vi "Equals.vi"(8 "error in (no error)":errorcluster caption="错误输入（无错误）", 10 "Point 输入":refnum<class "Point.lvclass"> caption="DNL_LabVIEW Object in", 11 "Point 输入":refnum<class "Point.lvclass"> caption="DNL_LabVIEW Object in") -> (0 "error out":errorcluster caption="错误输出", 2 "Equals":bool, 3 "Point 输出":refnum<class "Point.lvclass"> caption="DNL_LabVIEW Object out")   [LabVIEW 2011, in "Point.lvclass"]
uses:
  Point.lvclass
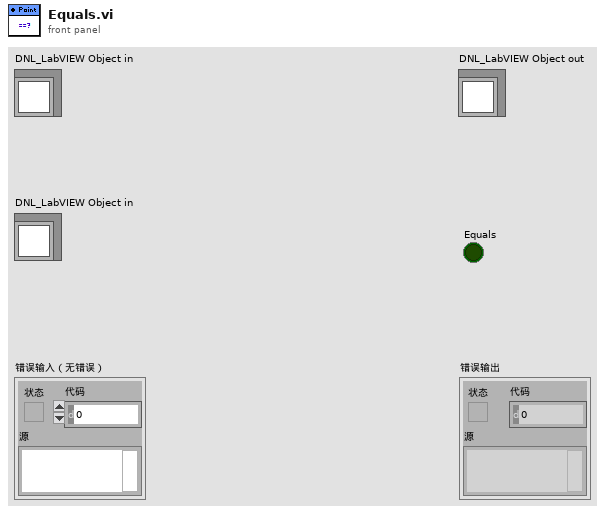
[diagram p1: front panel]
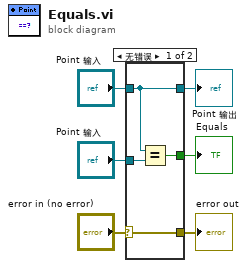
[diagram p0: block diagram]
diagram:
  n1 = case shown="无错误" "error in (no error)" {
    selector: "error in (no error)" -> [w10 w12]
    tunnel: [w10 w12] -> w5
    tunnel: [w8 w11] -> w3
    tunnel: "Point 输入" -> [w8 w11]
    tunnel: "Point 输入" -> [w9 _]
    tunnel: [w7 _] -> w1
    frame No Error {
      n2 = Equal?(x=w8, y=w9) -> (x = y?=w7:bool)
    }
    frame Error {
    }
  }
  "error out" <- w5
  "Point 输出" <- w3
  "Equals" <- w1
